vi "Irregular Array Subset (DBL, Index).vi"(8 "Indices":i32[](array[numeric]), 10 "Array":dbl[](array[numeric])) -> (0 "Indices (thru)":i32[](array[numeric]), 2 "Array Subset":dbl[](array[numeric]))   [LabVIEW 2020]
doc: "Extracts the values from the input array for which the corresponding boolean inputs are TRUE."
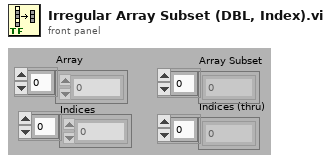
[diagram p1: front panel]
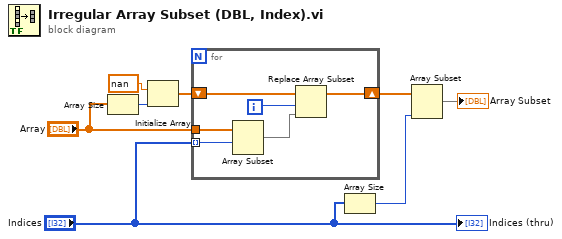
[diagram p0: block diagram]
diagram:
  n1 = Array Size(array="Array") -> (size(s)=w8:i32)
  n2 = Initialize Array(nan, w8) -> (w6:dbl[])
  n3 = for {
    tunnel: "Indices" -> [w9] mode=indexing
    shift-right: [w13] -> w4
    shift-left: w6 -> [w14]
    tunnel: "Array" -> [w12]
    i -> [w11]
    n4 = Array Subset(array=w12, index=w9) -> (w10:dbl[])  [unwired: 1 in]
    n5 = Replace Array Subset(array=w14, new element=w10, index=w11) -> (w13:dbl[])
  }
  n6 = Array Size(array="Indices") -> (size(s)=w1:i32)
  n7 = Array Subset(array=w4, length=w1) -> (→"Array Subset":dbl[])  [unwired: 1 in]
  "Indices (thru)" <- "Indices"
